vi "FRIC_navX_Internal_Serial_ProcessingLoop.vi"(9 "Stream Type":T1, 10 "Serial Port":T2, 11 "Update Rate (4Hz-100Hz)":u8=50 min=4 max=100) -> (0 "error out":errorcluster)   [LabVIEW 2015]
doc: "This navX VI handles the reading/writing for the navX. All of the good stuff is in here.\nTHIS VI SHOULD NOT BE CALLED BY THE USER!"
uses:
  navX Library v2/_TypeDefs/Z900_navX_DeviceTypeDef.ctl
  navX Library v2/_TypeDefs/Z900_navX_ProtocolTypeDef.ctl
  navX Library v2/_TypeDefs/Z900_navX_NotifyPacketTypeDef.ctl
  navX Library v2/_TypeDefs/Z900_navX_ActionTypeDef.ctl
  _NI WPI Serial USB/WPI_SerialPort_USB.ctl
  navX Library v2/_TypeDefs/Z900_navX_SerialStreamTypeDef.ctl
  TypeDefs/FRIC_navX_ProcessingLoopStatesTypeDef_I2C.ctl
  TypeDefs/FRIC_navX_I2C Process Loop TypeDef.ctl
  <vilib>/Rock Robotics/SystemInterfaces/Typedef/FPGA_TypedefDigitalModule.ctl
  <vilib>/Rock Robotics/SystemInterfaces/i2clib/i2c_bus.ctl
  navX Library v2/_TypeDefs/Z900_navX_IntegrationControlRegisters.ctl
  <vilib>/Rock Robotics/WPI/SPI/WPI_SPIDevRef.ctl
  <vilib>/Rock Robotics/SystemInterfaces/spilib/spi_bus.ctl
  <vilib>/Rock Robotics/WPI/SerialPort/WPI_SerialPortRef.ctl
  navX Library v2/_TypeDefs/Flags/Z900_navX_Flags_CapabilityTypeDef.ctl
  navX Library v2/_TypeDefs/Z900_navX_DeviceRegisters.ctl
  navX Library v2/_TypeDefs/navX Open TypeDefs/Z900_navX_OpenTypeDef_Serial.ctl
  navX Library v2/_Util/Encode Protocol/Z900_navX_Util_EncodeProtocol_SignedHundredths.vi
  navX Library v2/_Util/Encode Protocol/Z900_navX_Util_EncodeProtocol_UnsignedHundredths.vi
  navX Library v2/_Util/Encode Protocol/Z900_navX_Util_EncodeProtocol_UInt16.vi
  navX Library v2/Device/_Internal/SERIAL/Z900_navX_SERIAL_ValidatePacketChecksum.vi
  navX Library v2/Device/_Internal/SERIAL/Z900_navX_SERIAL_ValidatePacketTermination.vi
  navX Library v2/_Util/Encode Protocol/Z900_navX_Util_EncodeProtocol_Int16.vi
  navX Library v2/_Util/Z900_navX_Util_BigEndian_to_LittleEndian.vi
  <vilib>/Rock Robotics/SystemInterfaces/Utilities/FPGA_UtilitiesRead LocalTime.vi
  navX Library v2/navX Library v2.lvlib
  _NI WPI Serial USB/_NI WPI Serial USB.lvlib
panel:
  out "output cluster":T3={"Interface"={"Protocol"=enum."SERIAL", "Update Rate (4Hz-100Hz)"=4, "navX Open TypeDef"=variant}, "Notify Packet"=refnum, "Loop VI Refnum"=refnum, "Ready to Close Occurrence Refnum"=refnum, "Name"=""} {"Interface"."Update Rate (4Hz-100Hz)" min=4 max=60 step=1}
  out "Connected":bool
  in  "Halt":bool
  out "Registry":u8[](array[numeric])
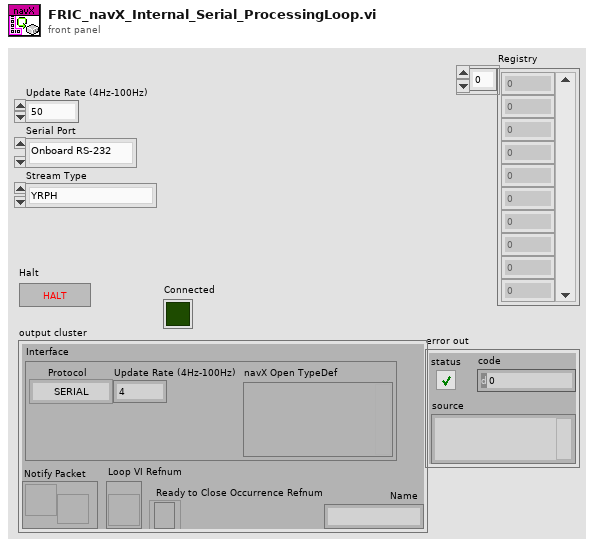
[diagram p1: front panel]
types:
  T1 = typedef "navX Library v2.lvlib/Z900_navX_SerialStreamTypeDef.ctl" = enum16{"YRPH", "Quaterinons", "Gyro/Raw", "AHRS", "AHRSAndPositioning"}
  T2 = typedef "_NI WPI Serial USB.lvlib/WPI_SerialPort_USB.ctl" = enum16{"Onboard RS-232", "MXP TTL", "USB"}
  T3 = typedef "navX Library v2.lvlib/Z900_navX_DeviceTypeDef.ctl" = cluster{"Interface":cluster{"Protocol":T4, "Update Rate (4Hz-100Hz)":u8, "navX Open TypeDef":variant}, "Notify Packet":refnum<notifier>, "Loop VI Refnum":refnum<vi>, "Ready to Close Occurrence Refnum":refnum<k4>, "Name":string}
  T4 = typedef "navX Library v2.lvlib/Z900_navX_ProtocolTypeDef.ctl" = enum16{"SERIAL", "I2C", "SPI"}
  T5 = typedef "FRIC_navX_ProcessingLoopStatesTypeDef_I2C.ctl" = enum16{"Process", "INI", "Check Packets Valid", "Close", "Decode Serial Packet", "Flush Serial", "Generate Command", "Last Packet Valid", "Open", "Read", "Reset Serial", "Set Termination Char", "Wait", "Write", "Exit"}
  T6 = typedef "FRIC_navX_I2C Process Loop TypeDef.ctl" = cluster{"State Array":T5[], "error":errorcluster, "FPGA Cluster":cluster{"Last Valid FPGA Time":dbl, "Error Count":i32, "Initialized":bool}, "Device Info":T3, "I2CDevRef":cluster{"DevStatus":errorcluster, "Controller":T7, "Device Address":u8, "Handle":i32, "I2C Bus":T8}, "Registry":u8[], "Command Array":T9[], "Connected?":bool, "navX Device Memory Size":i32, "notification":T10, "Memory Size Set":bool, "SPIDevRef":T12, "navX Serial Open":cluster{"Serial Port":T2, "Stream Type":T1}, "SerialPortRef":T14, "Serial Read Buffer":string, "Serial Write Buffer":string[]}
  T7 = typedef "FPGA_TypedefDigitalModule.ctl" = enum16{"Controller 1"}
  T8 = typedef "i2c_bus.ctl" = enum16{"I2C On-Board", "I2C MXP", "Invalid"}
  T9 = typedef "navX Library v2.lvlib/Z900_navX_IntegrationControlRegisters.ctl" = u8
  T10 = typedef "navX Library v2.lvlib/Z900_navX_NotifyPacketTypeDef.ctl" = cluster{"navX Action":T11, "Data":variant}
  T11 = typedef "navX Library v2.lvlib/Z900_navX_ActionTypeDef.ctl" = enum16{"None", "Halt", "Normal Read", "Update Serial Protocol", "Update Rate Htz", "Zero-Yaw", "Zero-Displacement", "Zero-Velocity"}
  T12 = typedef "WPI_SPIDevRef.ctl" = cluster{"DevStatus":errorcluster, "Handle":i32, "Controller":T7, "SPI Bus":T13}
  T13 = typedef "spi_bus.ctl" = enum16{"SPI On-Board, CS0", "SPI On-Board, CS1", "SPI On-Board, CS2", "SPI On-Board, CS3", "SPI MXP", "Invalid"}
  T14 = typedef "WPI_SerialPortRef.ctl" = cluster{"DevStatus":errorcluster, "Serial Port Name":refnum<visa-resource-name>}
  T15 = typedef "navX Library v2.lvlib/Z900_navX_OpenTypeDef_Serial.ctl" = cluster{"Serial Port":T2, "Stream Type":T1}
  T16 = typedef "navX Library v2.lvlib/Z900_navX_DeviceRegisters.ctl" = u8
  T17 = typedef "navX Library v2.lvlib/Z900_navX_Flags_CapabilityTypeDef.ctl" = u16
  T18 = cluster{"Last Valid FPGA Time":dbl, "Error Count":i32, "Initialized":bool}
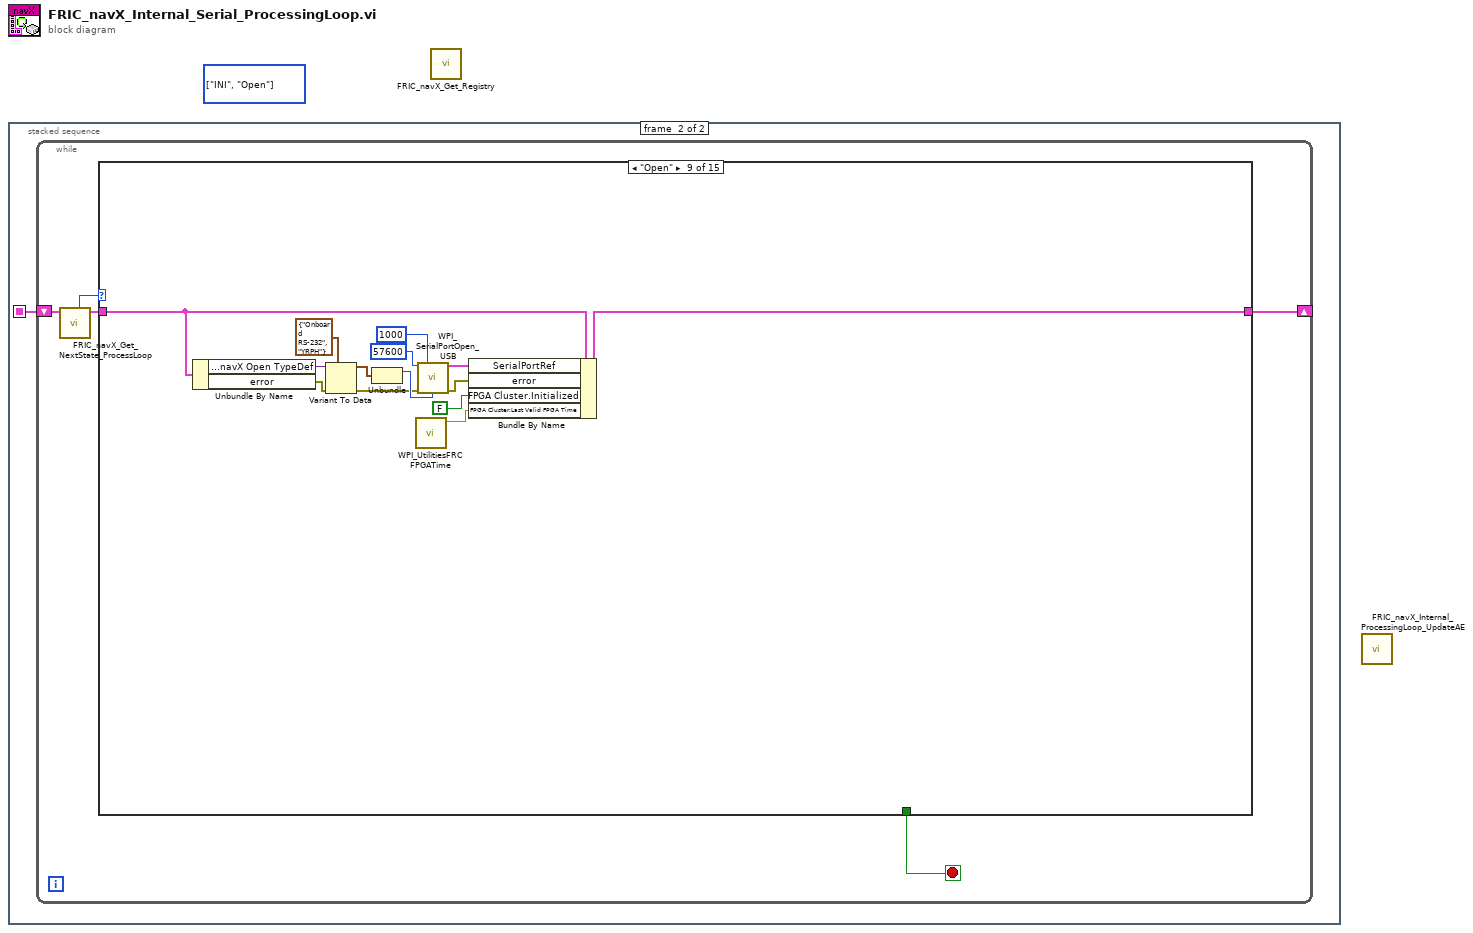
[diagram p0: block diagram]
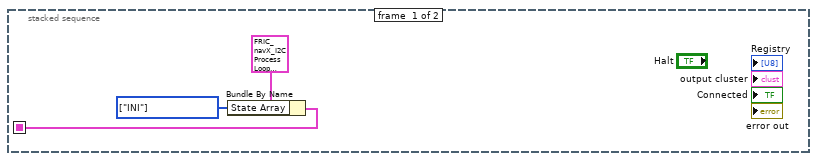
[diagram p2: hidden frame]
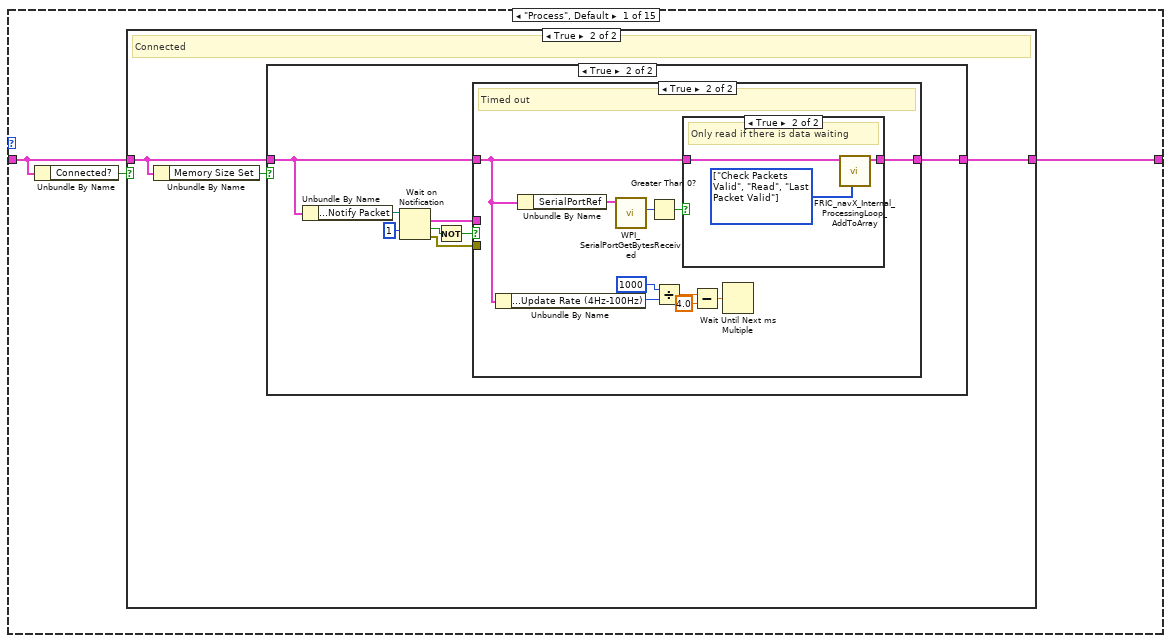
[diagram p3: hidden frame]
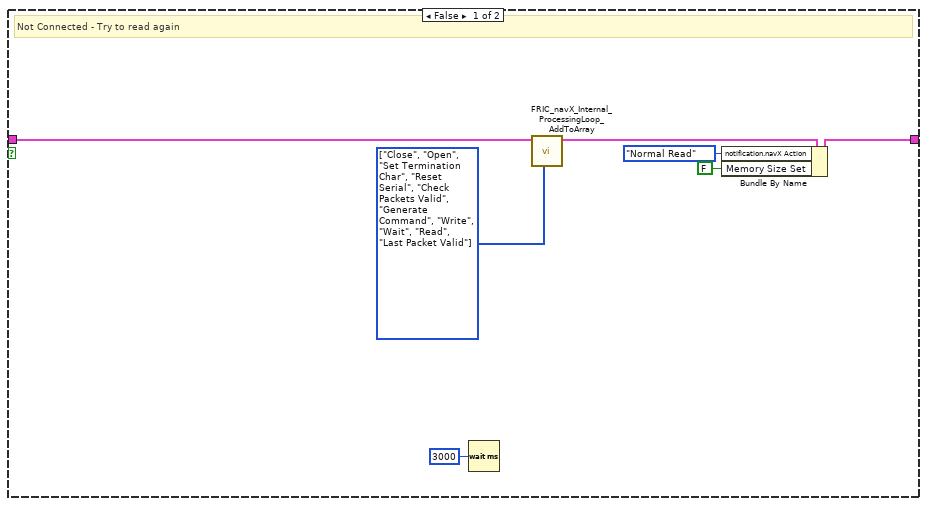
[diagram p4: hidden frame]
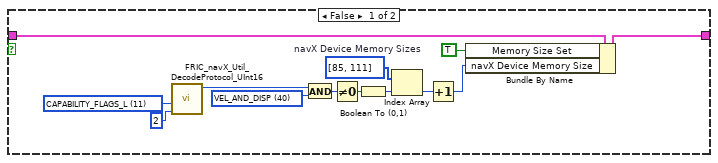
[diagram p5: hidden frame]
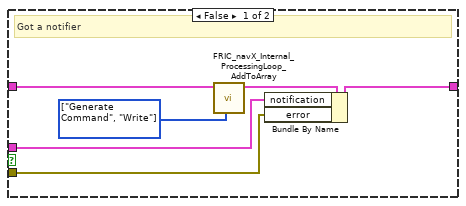
[diagram p6: hidden frame]
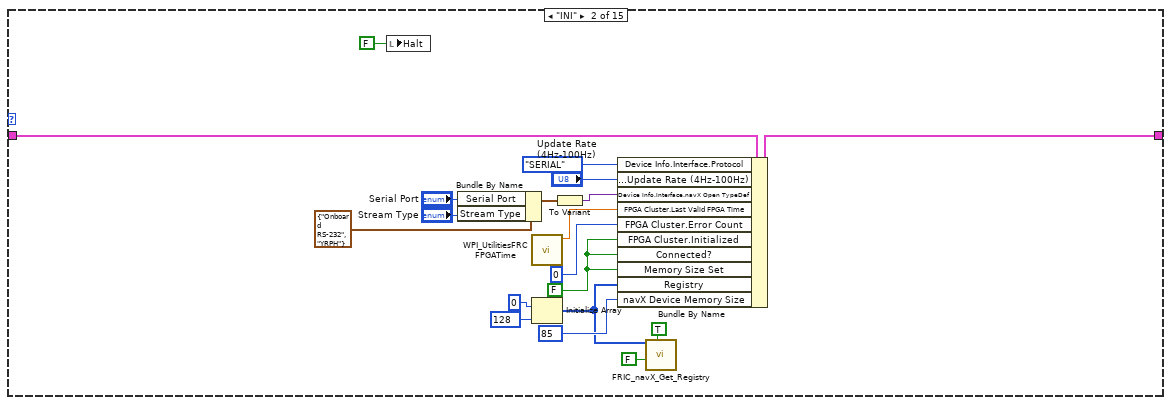
[diagram p8: hidden frame]
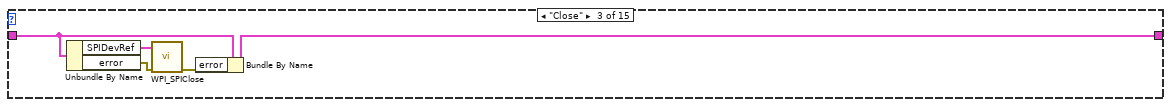
[diagram p9: hidden frame]
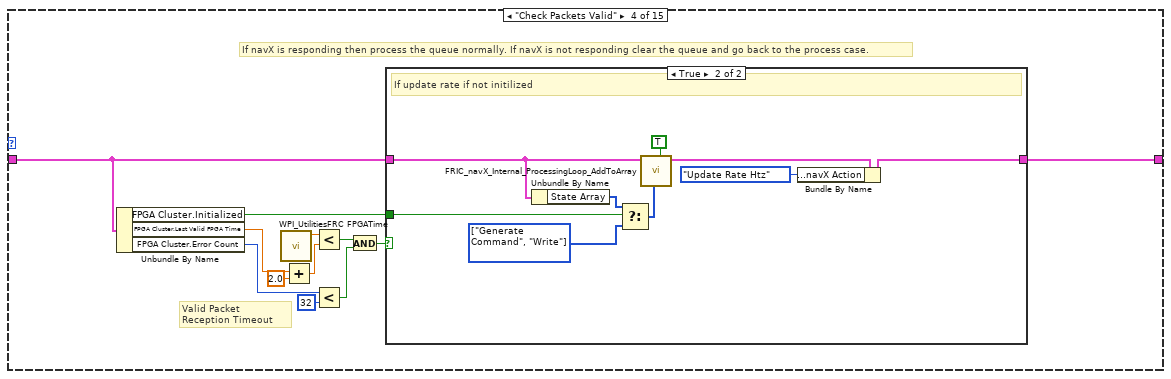
[diagram p10: hidden frame]
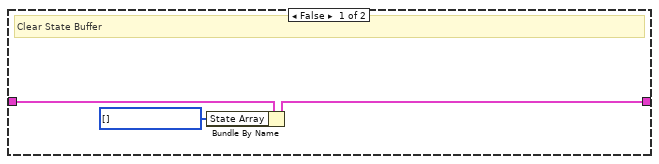
[diagram p11: hidden frame]
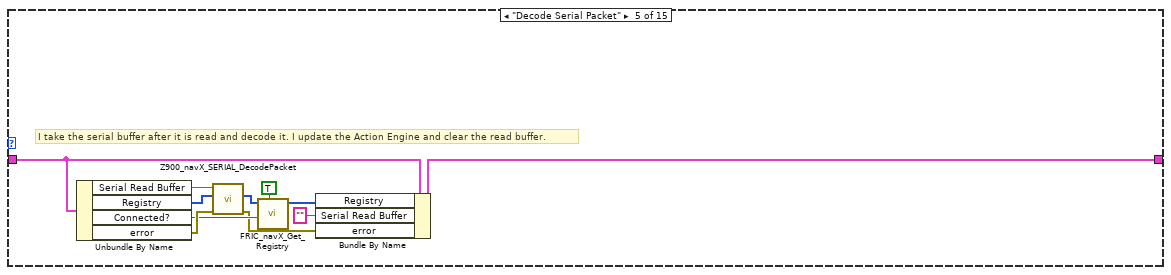
[diagram p12: hidden frame]
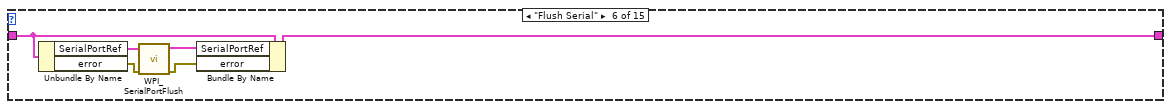
[diagram p13: hidden frame]
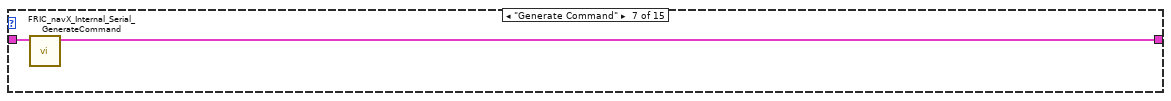
[diagram p14: hidden frame]
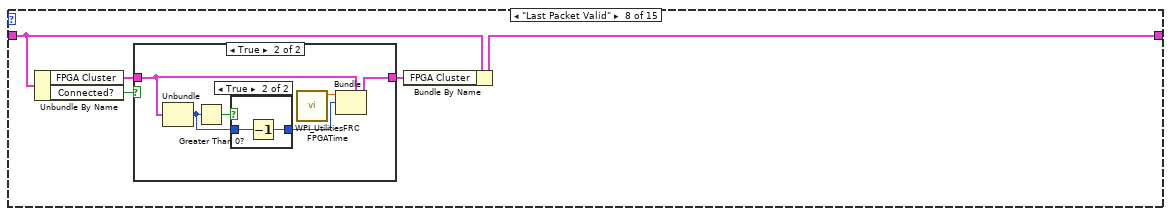
[diagram p15: hidden frame]
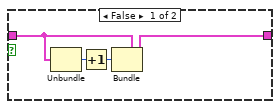
[diagram p16: hidden frame]
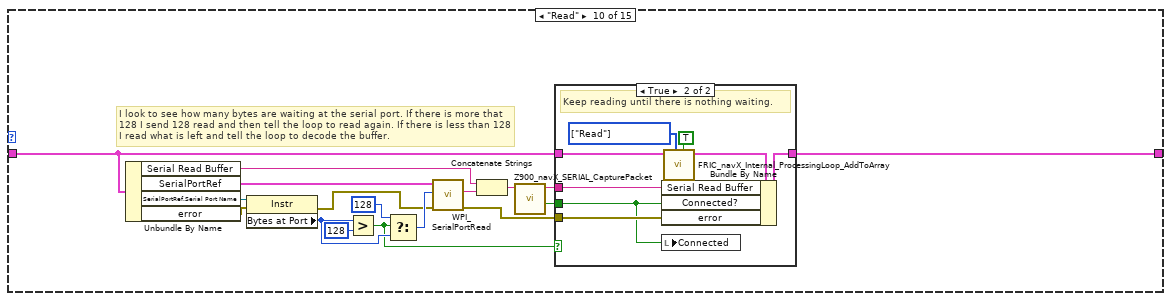
[diagram p18: hidden frame]
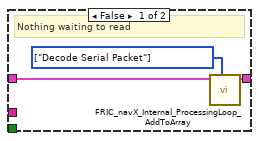
[diagram p19: hidden frame]
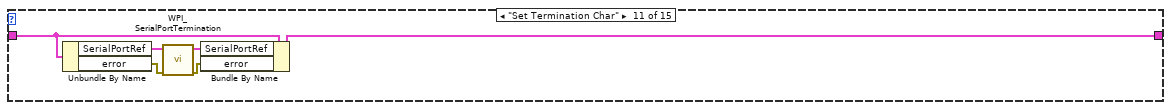
[diagram p20: hidden frame]
diagram:
  (unwired) T5[] [enum."INI", enum."Open"] items=["Process", "INI", "Check Packets Valid", "Close", "Decode Serial Packet", "Flush Serial", "Generate Command", "Last Packet Valid", "Open", "Read", "Reset Serial", "Set Termination Char", "Wait", "Write", "Exit"]
  n1 = stacked-sequence {
    seq-local: [w3 _] -> [_ w4]
    frame #0 {
      w1 = T5[] [enum."INI"] items=["Process", "INI", "Check Packets Valid", "Close", "Decode Serial Packet", "Flush Serial", "Generate Command", "Last Packet Valid", "Open", "Read", "Reset Serial", "Set Termination Char", "Wait", "Write", "Exit"] ("State Array")
      n2 = Bundle By Name(cluster=T6 {"State Array"=[enum."INI", enum."Open"], "error"={"status"=FALSE, "code"=0, "source"=""}, "FPGA Cluster"={"Last Valid FPGA Time"=0.0, "Error Count"=0, "Initialized"=FALSE}, "Device Info"={"Interface"={"Protocol"=enum."SERIAL", "Update Rate (4Hz-100Hz)"=4, "navX Open TypeDef"=variant}, "Notify Packet"=refnum, "Loop VI Refnum"=refnum, "Ready to Close Occurrence Refnum"=refnum, "Name"=""}, "I2CDevRef"={"DevStatus"={"status"=FALSE, "code"=0, "source"=""}, "Controller"=enum."Controller 1", "Device Address"=0, "Handle"=0, "I2C Bus"=enum."Invalid"}, "Registry"=[], "Command Array"=[214, 32], "Connected?"=FALSE, "navX Device Memory Size"=85, "notification"={"navX Action"=enum."None", "Data"=variant}, "Memory Size Set"=FALSE, "SPIDevRef"={"DevStatus"={"status"=FALSE, "code"=0, "source"=""}, "Handle"=0, "Controller"=enum."Controller 1", "SPI Bus"=enum."SPI On-Board, CS0"}, "navX Serial Open"={"Serial Port"=enum."Onboard RS-232", "Stream Type"=enum."YRPH"}, "SerialPortRef"={"DevStatus"={"status"=FALSE, "code"=0, "source"=""}, "Serial Port Name"=""}, "Serial Read Buffer"="", "Serial Write Buffer"=[]} ("I2C Process Loop TypeDef"), "State Array"=w1) -> (w3:T6)
    }
    frame #1 {
      n3 = while {
        shift-right: [w5] -> _
        shift-left: w4 -> [w8]
        stop <- w9 stop-if-true
        n4 = call "FRIC_navX_Get_NextState_ProcessLoop.vi"("I2C Process Loop TypeDef (in)"=w8) -> ("I2C Process Loop TypeDef (out)"=w7:T6, "Current State"=w6:T5)  [unwired: 9 in]
        n5 = case shown="\"Open\"" w6 {
          tunnel: [_ _ _ _ _ _ _ _ _ _ _ _ _ _ TRUE] -> w9
          tunnel: w7 -> [w10 w78 w87 w91 w117 w124 w130 w134 w160 w167 w191 w201 w204 w219 w226]
          tunnel: [w12 w72 w86 w92 w116 w123 w129 w133 w159 w166 w192 w202 w204 w207 w226] -> w5
          frame "Process", Default {
            n6 = Unbundle By Name(w10) -> ("Connected?"=w11:bool)
            n7 = case shown="True" w11 {
              tunnel: w10 -> [w18 w21]
              tunnel: [w15 w22] -> w12
              frame False {
                w17 = T5[] [enum."Close", enum."Open", enum."Set Termination Char", enum."Reset Serial", enum."Check Packets Valid", enum."Generate Command", enum."Write", enum."Wait", enum."Read", enum."Last Packet Valid"] items=["Process", "INI", "Check Packets Valid", "Close", "Decode Serial Packet", "Flush Serial", "Generate Command", "Last Packet Valid", "Open", "Read", "Reset Serial", "Set Termination Char", "Wait", "Write", "Exit"]
                # "Not Connected - Try to read again"
                n8 = Wait (ms)(milliseconds to wait=u32 3000) -> ()  [unwired: 1 out]
                n9 = call "FRIC_navX_Internal_ProcessingLoop_AddToArray.vi"("States Array"=w17, "I2C Process Loop TypeDef (in)"=w18) -> ("I2C Process Loop TypeDef (out)"=w16:T6)  [unwired: 9 in]
                n10 = Bundle By Name(cluster=w16, "notification.navX Action"=Z900_navX_ActionTypeDef."Normal Read", "Memory Size Set"=FALSE) -> (w15:T6)
              }
              frame True {
                # "Connected"
                n11 = Unbundle By Name(w21) -> ("Memory Size Set"=w20:bool)
                n12 = case shown="True" w20 {
                  tunnel: [w34 w40] -> w22
                  tunnel: w21 -> [w35 w36]
                  frame False {
                    w33 = T16 11 items=["WHOAMI"=0, "HW_REV"=1, "FW_VER_MAJOR"=2, "FW_VER_MINOR"=3, "UPDATE_RATE_HZ"=4, "ACCEL_FSR_G"=5, "GYRO_FSR_DPS"=6, "OP_STATUS"=8, "CAL_STATUS"=9, "SELFTEST_STATUS"=10, "CAPABILITY_FLAGS_L"=11, "CAPABILITY_FLAGS_H"=12, "SENSOR_STATUS"=16, "TIMESTAMP"=18, "YAW"=22, "ROLL"=24, "PITCH"=26, "HEADING"=28, "FUSED_HEADING"=30, "ALTITUDE_I"=32, "ALTITUDE_D"=34, "LINERA_ACC_X"=36, "LINERA_ACC_Y"=38, "LINERA_ACC_Z"=40, "QUAT_W"=42, "QUAT_X"=44, "QUAT_Y"=46, "QUAT_Z"=48, "MPU_TEMP_C"=50, "GYRO_X"=52, "GYRO_Y"=54, "GYRO_Z"=56, "ACC_X"=58, "ACC_Y"=60, "ACC_Z"=62, "MAG_X"=64, "MAG_Y"=66, "MAG_Z"=68, "PRESSURE_I"=70, "PRESSURE_D"=72, "PRESSURE_TEMP"=74, "YAW_OFFSET"=76, "QUAT_OFFSET_W"=78, "QUAT_OFFSET_X"=80, "QUAT_OFFSET_Y"=82, "QUAT_OFFSET_Z"=84, "INTEGRATION_CONTROL"=86, "VELOCITY_X"=88, "VELOCITY_Y"=92, "VELOCITY_Z"=96, "DISPLACMENT_X"=100, "DISPLACMENT_Y"=104, "DISPLACEMENT_Z"=108] ("Device Register")
                    w28 = T17 40 items=["OMNIMOUNT"=4, "OMNIMOUNT_CONFIG_MASK"=38, "VEL_AND_DISP"=40, "YAW_RESET"=80] ("Capability Flag")
                    w29 = i32[] [85, 111]  # navX Device Memory Sizes
                    n13 = call "FRIC_navX_Util_DecodeProtocol_UInt16.vi"("length"=2, "Device Register"=w33) -> ("Value"=w26:u16)  [unwired: 9 in]
                    n14 = And(x=w26, y=w28) -> (x .and. y?=w27:T17)
                    n15 = Not Equal To 0?(x=w27) -> (x != 0?=w30:bool)
                    n16 = Boolean To (0,1)(Boolean=w30) -> (0, 1=w31:i16)
                    n17 = Index Array(array=w29, index=w31) -> (element=w24:i32)
                    n18 = Increment(x=w24) -> (x+1=w23:i32)
                    n19 = Bundle By Name(cluster=w35, "Memory Size Set"=TRUE, "navX Device Memory Size"=w23) -> (w34:T6)
                  }
                  frame True {
                    n20 = Unbundle By Name(w36) -> ("Device Info.Notify Packet"=w43:refnum<notifier>)
                    n21 = Wait on Notification(notifier=w43, timeout in ms (-1)=1) -> (notification=w38:T10, timed out?=w41:bool, error out=w37:errorcluster)  [unwired: 2 in, 1 out]
                    n22 = Not(x=w41) -> (.not. x?=w39:bool)
                    n23 = case shown="True" w39 {
                      tunnel: w36 -> [w49 w53]
                      tunnel: [w48 w54] -> w40
                      tunnel: w38 -> [w47 _]
                      tunnel: w37 -> [w44 _]
                      frame False {
                        w45 = T5[] [enum."Generate Command", enum."Write"] items=["Process", "INI", "Check Packets Valid", "Close", "Decode Serial Packet", "Flush Serial", "Generate Command", "Last Packet Valid", "Open", "Read", "Reset Serial", "Set Termination Char", "Wait", "Write", "Exit"] ("States Array")
                        # "Got a notifier"
                        n24 = call "FRIC_navX_Internal_ProcessingLoop_AddToArray.vi"("States Array"=w45, "I2C Process Loop TypeDef (in)"=w49) -> ("I2C Process Loop TypeDef (out)"=w46:T6)  [unwired: 9 in]
                        n25 = Bundle By Name(cluster=w46, "notification"=w47, "error"=w44) -> (w48:T6)
                      }
                      frame True {
                        # "Timed out"
                        n26 = Unbundle By Name(w53) -> ("Device Info.Interface.Update Rate (4Hz-100Hz)"=w59:u8)
                        n27 = Unbundle By Name(w53) -> ("SerialPortRef"=w52:T14)
                        n28 = call <vilib>:"WPI_SerialPortGetBytesReceived.vi"("SerialPortRef"=w52) -> ("Bytes at Port"=w51:u32)  [unwired: 8 in, 2 out]
                        n29 = Greater Than 0?(x=w51) -> (x > 0?=w50:bool)
                        n30 = Divide(x=i16 1000, y=w59) -> (x/y=w57:dbl)
                        n31 = case shown="True" w50 {
                          tunnel: [w60 w62] -> w54
                          tunnel: w53 -> [w60 w61]
                          frame False {
                          }
                          frame True {
                            w63 = T5[] [enum."Check Packets Valid", enum."Read", enum."Last Packet Valid"] items=["Process", "INI", "Check Packets Valid", "Close", "Decode Serial Packet", "Flush Serial", "Generate Command", "Last Packet Valid", "Open", "Read", "Reset Serial", "Set Termination Char", "Wait", "Write", "Exit"]
                            # "Only read if there is data waiting"
                            n32 = call "FRIC_navX_Internal_ProcessingLoop_AddToArray.vi"("States Array"=w63, "I2C Process Loop TypeDef (in)"=w61) -> ("I2C Process Loop TypeDef (out)"=w62:T6)  [unwired: 9 in]
                          }
                        }
                        n33 = Subtract(x=w57, y=4.0) -> (x-y=w55:dbl)
                        n34 = Wait Until Next ms Multiple(millisecond multiple=w55) -> ()  [unwired: 1 out]
                      }
                    }
                  }
                }
              }
            }
          }
          frame "INI" {
            w70 = FALSE ("Initialized")
            n35 = local write "Halt"(FALSE ("Halt")) -> ()
            n36 = Bundle By Name(cluster=T15 {"Serial Port"=enum."Onboard RS-232", "Stream Type"=enum."YRPH"} ("navX Serial Open"), "Serial Port"="Serial Port", "Stream Type"="Stream Type") -> (w79:T15)
            n37 = call <vilib>:"WPI_UtilitiesFRC FPGATime.vi"() -> ("FPGA Time"=w74:dbl)  [unwired: 10 in, 1 out]
            n38 = Initialize Array(u8 0 ("Received Data"), 128 ("hex")) -> (w68:u8[])
            n39 = To Variant(anything=w79) -> (Variant=w75:variant)
            n40 = Bundle By Name(cluster=w78, "Device Info.Interface.Protocol"=Z900_navX_ProtocolTypeDef."SERIAL" ("Protocol"), "Device Info.Interface.Update Rate (4Hz-100Hz)"="Update Rate (4Hz-100Hz)", "Device Info.Interface.navX Open TypeDef"=w75, "FPGA Cluster.Last Valid FPGA Time"=w74, "FPGA Cluster.Error Count"=0 ("Error Count"), "FPGA Cluster.Initialized"=w70, "Connected?"=w70, "Memory Size Set"=w70, "Registry"=w68, "navX Device Memory Size"=85 ("hex")) -> (w72:T6)
            n41 = call "FRIC_navX_Get_Registry.vi"("Update"=TRUE, "Connected?"=FALSE, "Registry (in)"=w68) -> ()  [unwired: 7 in, 2 out]
          }
          frame "Close" {
            n42 = Unbundle By Name(w87) -> ("SPIDevRef"=w85:T12, "error"=w84:errorcluster)
            n43 = call <vilib>:"WPI_SPIClose.vi"("error in (no error)"=w84, "SPIDevRef"=w85) -> ("error out"=w83:errorcluster)  [unwired: 9 in]
            n44 = Bundle By Name(cluster=w87, "error"=w83) -> (w86:T6)
          }
          frame "Check Packets Valid" {
            # "If navX is responding then process the queue normally. If navX is not responding clear the queue and go back to the process case."
            # "Valid Packet Reception Timeout"
            n45 = Unbundle By Name(w91) -> ("FPGA Cluster.Initialized"=w89:bool, "FPGA Cluster.Last Valid FPGA Time"=w90:dbl, "FPGA Cluster.Error Count"=w88:i32)
            n46 = call <vilib>:"WPI_UtilitiesFRC FPGATime.vi"() -> ("FPGA Time"=w97:dbl)  [unwired: 10 in, 1 out]
            n47 = Add(x=w90, y=2.0) -> (x+y=w98:dbl)
            n48 = Less?(x=w97, y=w98) -> (x < y?=w95:bool)
            n49 = Less?(x=w88, y=32) -> (x < y?=w94:bool)
            n50 = And(x=w95, y=w94) -> (x .and. y?=w93:bool)
            n51 = case shown="True" w93 {
              tunnel: w91 -> [w102 w109]
              tunnel: [w101 w104] -> w92
              tunnel: w89 -> [_ w110]
              frame False {
                w100 = T5[] [] items=["Process", "INI", "Check Packets Valid", "Close", "Decode Serial Packet", "Flush Serial", "Generate Command", "Last Packet Valid", "Open", "Read", "Reset Serial", "Set Termination Char", "Wait", "Write", "Exit"] ("f")
                # "Clear State Buffer"
                n52 = Bundle By Name(cluster=w102, "State Array"=w100) -> (w101:T6)
              }
              frame True {
                w106 = T5[] [enum."Generate Command", enum."Write"] items=["Process", "INI", "Check Packets Valid", "Close", "Decode Serial Packet", "Flush Serial", "Generate Command", "Last Packet Valid", "Open", "Read", "Reset Serial", "Set Termination Char", "Wait", "Write", "Exit"] ("f")
                # "If update rate if not initilized"
                n53 = Unbundle By Name(w109) -> ("State Array"=w108:T5[])
                n54 = Select(t=w108, s=w110, f=w106) -> (s? t:f=w107:T5[])
                n55 = call "FRIC_navX_Internal_ProcessingLoop_AddToArray.vi"("Add to beginning"=TRUE, "States Array"=w107, "I2C Process Loop TypeDef (in)"=w109) -> ("I2C Process Loop TypeDef (out)"=w105:T6)  [unwired: 8 in]
                n56 = Bundle By Name(cluster=w105, "notification.navX Action"=Z900_navX_ActionTypeDef."Update Rate Htz") -> (w104:T6)
              }
            }
          }
          frame "Decode Serial Packet" {
            # "I take the serial buffer after it is read and decode it. I update the Action Engine and clear the read buffer."
            n57 = Unbundle By Name(w117) -> ("Serial Read Buffer"=w120:string, "Registry"=w119:u8[], "Connected?"=w113:bool, "error"=w114:errorcluster)
            n58 = call "Z900_navX_SERIAL_DecodePacket.vi"("error in (no error)"=w114, "Data"=w119, "Packet"=w120) -> ("error out"=w112:errorcluster, "Data"=w118:u8[])  [unwired: 6 in, 1 out]
            n59 = call "FRIC_navX_Get_Registry.vi"("Update"=TRUE, "Connected?"=w113, "Registry (in)"=w118) -> ("Registry (out)"=w121:u8[])  [unwired: 7 in, 1 out]
            n60 = Bundle By Name(cluster=w117, "Registry"=w121, "Serial Read Buffer"="", "error"=w112) -> (w116:T6)
          }
          frame "Flush Serial" {
            n61 = Unbundle By Name(w124) -> ("SerialPortRef"=w128:T14, "error"=w127:errorcluster)
            n62 = call <vilib>:"WPI_SerialPortFlush.vi"("error in (no error)"=w127, "SerialPortRef"=w128) -> ("error out"=w125:errorcluster, "SerialPortRef"=w126:T14)  [unwired: 8 in]
            n63 = Bundle By Name(cluster=w124, "SerialPortRef"=w126, "error"=w125) -> (w123:T6)
          }
          frame "Generate Command" {
            n64 = call "FRIC_navX_Internal_Serial_GenerateCommand.vi"("I2C Process Loop TypeDef (in)"=w130) -> ("I2C Process Loop TypeDef (out)"=w129:T6)  [unwired: 10 in]
          }
          frame "Last Packet Valid" {
            n65 = Unbundle By Name(w134) -> ("FPGA Cluster"=w135:T18, "Connected?"=w131:bool)
            n66 = case shown="True" w131 {
              tunnel: [w138 w145] -> w132
              tunnel: w135 -> [w137 w141]
              frame False {
                n67 = Unbundle(w137) -> ("Error Count"=w136:i32)  [unwired: 2 out]
                n68 = Increment(x=w136) -> (x+1=w139:i32)
                n69 = Bundle(cluster=w137, "Error Count"=w139) -> (w138:T18)  [unwired: 2 in]
              }
              frame True {
                n70 = Unbundle(w141) -> ("Error Count"=w140:i32)  [unwired: 2 out]
                n71 = Greater Than 0?(x=w140) -> (x > 0?=w143:bool)
                n72 = case shown="True" w143 {
                  tunnel: [w146 w148] -> w142
                  tunnel: w140 -> [w146 w147]
                  frame False {
                  }
                  frame True {
                    n73 = Decrement(x=w147) -> (x-1=w148:i32)
                  }
                }
                n74 = call <vilib>:"WPI_UtilitiesFRC FPGATime.vi"() -> ("FPGA Time"=w144:dbl)  [unwired: 10 in, 1 out]
                n75 = Bundle(cluster=w141, "Last Valid FPGA Time"=w144, "Error Count"=w142) -> (w145:T18)  [unwired: 1 in]
              }
            }
            n76 = Bundle By Name(cluster=w134, "FPGA Cluster"=w132) -> (w133:T6)
          }
          frame "Open" {
            n77 = Unbundle By Name(w160) -> ("Device Info.Interface.navX Open TypeDef"=w162:variant, "error"=w158:errorcluster)
            n78 = Variant To Data(error in=w158, type=T15 {"Serial Port"=enum."Onboard RS-232", "Stream Type"=enum."YRPH"} ("navX Serial Open"), Variant=w162) -> (data=w161:T15, error out=w152:errorcluster)
            n79 = Unbundle(w161) -> ("Serial Port"=w153:T2)  [unwired: 1 out]
            n80 = call <vilib>:"WPI_UtilitiesFRC FPGATime.vi"() -> ("FPGA Time"=w149:dbl)  [unwired: 10 in, 1 out]
            n81 = call "WPI_SerialPortOpen_USB.vi"("Baud Rate"=u32 57600, "Timeout Value (ms)"=u32 1000, "error in (no error)"=w152, "Serial Port"=w153) -> ("SerialPortRef"=w150:T14, "error out"=w151:errorcluster)  [unwired: 10 in]
            n82 = Bundle By Name(cluster=w160, "SerialPortRef"=w150, "error"=w151, "FPGA Cluster.Initialized"=FALSE ("Initialized"), "FPGA Cluster.Last Valid FPGA Time"=w149) -> (w159:T6)
          }
          frame "Read" {
            # "I look to see how many bytes are waiting at the serial port. If there is more that 128 I send 128 read and then tell the loop to read again. If there is less than 128 I read what is left and tell the loop to decode the buffer."
            n83 = Unbundle By Name(w167) -> ("Serial Read Buffer"=w175:string, "SerialPortRef"=w176:T14, "SerialPortRef.Serial Port Name"=w179:refnum<visa-resource-name>, "error"=w178:errorcluster)
            n84 = property class="Instr"(reference=w179, error in=w178) -> (error out=w169:errorcluster, "Bytes at Port"=w172:u32)  [unwired: 1 in]
            n85 = Greater?(x=w172, y=u32 128) -> (0:w168:bool)
            n86 = Select(t=u32 128 ("y"), s=w168, f=w172) -> (s? t:f=w170:u32)
            n87 = call <vilib>:"WPI_SerialPortRead.vi"("error in (no error)"=w169, "Num Bytes to Read"=w170, "SerialPortRef"=w176) -> ("error out"=w163:errorcluster, "Buffer"=w177:string)  [unwired: 6 in, 1 out]
            n88 = Concatenate Strings(w175, w177) -> (w174:string)
            n89 = call "Z900_navX_SERIAL_CapturePacket.vi"("Buffer"=w174) -> ("Packet Located"=w164:bool, "Buffer"=w165:string)  [unwired: 7 in, 2 out]
            n90 = case shown="True" w168 {
              tunnel: w167 -> [w182 w190]
              tunnel: [w181 w186] -> w166
              tunnel: w165 -> [_ w185]
              tunnel: w164 -> [_ w183]
              tunnel: w163 -> [_ w184]
              frame False {
                w180 = T5[] [enum."Decode Serial Packet"] items=["Process", "INI", "Check Packets Valid", "Close", "Decode Serial Packet", "Flush Serial", "Generate Command", "Last Packet Valid", "Open", "Read", "Reset Serial", "Set Termination Char", "Wait", "Write", "Exit"] ("States Array")
                # "Nothing waiting to read"
                n91 = call "FRIC_navX_Internal_ProcessingLoop_AddToArray.vi"("States Array"=w180, "I2C Process Loop TypeDef (in)"=w182) -> ("I2C Process Loop TypeDef (out)"=w181:T6)  [unwired: 9 in]
              }
              frame True {
                w189 = T5[] [enum."Read"] items=["Process", "INI", "Check Packets Valid", "Close", "Decode Serial Packet", "Flush Serial", "Generate Command", "Last Packet Valid", "Open", "Read", "Reset Serial", "Set Termination Char", "Wait", "Write", "Exit"] ("States Array")
                # "Keep reading until there is nothing waiting."
                n92 = local write "Connected"(w183) -> ()
                n93 = call "FRIC_navX_Internal_ProcessingLoop_AddToArray.vi"("Add to beginning"=TRUE, "States Array"=w189, "I2C Process Loop TypeDef (in)"=w190) -> ("I2C Process Loop TypeDef (out)"=w187:T6)  [unwired: 8 in]
                n94 = Bundle By Name(cluster=w187, "Serial Read Buffer"=w185, "Connected?"=w183, "error"=w184) -> (w186:T6)
              }
            }
          }
          frame "Set Termination Char" {
            n95 = Unbundle By Name(w191) -> ("SerialPortRef"=w196:T14, "error"=w195:errorcluster)
            n96 = call <vilib>:"WPI_SerialPortTermination.vi"("error in (no error)"=w195, "SerialPortRef"=w196) -> ("error out"=w193:errorcluster, "SerialPortRef"=w194:T14)  [unwired: 8 in]
            n97 = Bundle By Name(cluster=w191, "SerialPortRef"=w194, "error"=w193) -> (w192:T6)
          }
          frame "Reset Serial" {
            n98 = Unbundle By Name(w201) -> ("SerialPortRef"=w200:T14, "error"=w198:errorcluster)
            n99 = call <vilib>:"WPI_SerialPortReset.vi"("error in (no error)"=w198, "SerialPortRef"=w200) -> ("error out"=w197:errorcluster, "SerialPortRef"=w199:T14)  [unwired: 8 in]
            n100 = Bundle By Name(cluster=w201, "SerialPortRef"=w199, "error"=w197) -> (w202:T6)
          }
          frame "Wait" {
            n101 = Wait (ms)(milliseconds to wait=u32 1) -> ()  [unwired: 1 out]
          }
          frame "Write" {
            w206 = T5[] [enum."Flush Serial"] items=["Process", "INI", "Check Packets Valid", "Close", "Decode Serial Packet", "Flush Serial", "Generate Command", "Last Packet Valid", "Open", "Read", "Reset Serial", "Set Termination Char", "Wait", "Write", "Exit"] ("States Array")
            # "This adds a flush after any write so we don't always have to tell the array to flush."
            n102 = Unbundle By Name(w219) -> ("SerialPortRef"=w217:T14, "Serial Write Buffer"=w214:string[], "SerialPortRef.DevStatus"=w218:errorcluster)
            n103 = Delete From Array(array=w214, index=0) -> (deleted portion=w213:string, array with subset deleted=w210:string[])  [unwired: 1 in]
            n104 = call <vilib>:"WPI_SerialPortWrite.vi"("error in (no error)"=w218, "Buffer"=w213, "SerialPortRef"=w217) -> ("error out"=w216:errorcluster, "SerialPortRef"=w215:T14)  [unwired: 6 in, 1 out]
            n105 = Empty Array?(array=w210) -> (empty?=w209:bool)
            n106 = Bundle By Name(cluster=w219, "SerialPortRef"=w215, "error"=w216, "Serial Write Buffer"=w210) -> (w211:T6)
            n107 = case shown="False" w209 {
              tunnel: [w223 w224] -> w208
              tunnel: w211 -> [w222 w224]
              frame False {
                w221 = T5[] [enum."Write"] items=["Process", "INI", "Check Packets Valid", "Close", "Decode Serial Packet", "Flush Serial", "Generate Command", "Last Packet Valid", "Open", "Read", "Reset Serial", "Set Termination Char", "Wait", "Write", "Exit"] ("States Array")
                # "Write again because buffer is not empty."
                n108 = call "FRIC_navX_Internal_ProcessingLoop_AddToArray.vi"("Add to beginning"=TRUE, "States Array"=w221, "I2C Process Loop TypeDef (in)"=w222) -> ("I2C Process Loop TypeDef (out)"=w223:T6)  [unwired: 8 in]
              }
              frame True {
                # "Process the rest of the state array"
              }
            }
            n109 = call "FRIC_navX_Internal_ProcessingLoop_AddToArray.vi"("Add to beginning"=TRUE, "States Array"=w206, "I2C Process Loop TypeDef (in)"=w208) -> ("I2C Process Loop TypeDef (out)"=w207:T6)  [unwired: 8 in]
          }
          frame "Exit" {
            n110 = Unbundle By Name(w226) -> ("Device Info"=w225:T3)
            n111 = in-place {
              in-place-border: [TRUE] -> w228
              in-place-border: w225 -> [w229]
              # "Set Occurence of Close"
              n112 = Unbundle By Name(w229) -> ("Ready to Close Occurrence Refnum"=w231:refnum<k4>)
              n113 = local write "Halt"(FALSE ("Halt")) -> ()
              n114 = Set Occurrence(w231) -> ()
            }
            n115 = Stop(stop? (T)=w228) -> ()
          }
        }
      }
    }
  }
  n116 = call "FRIC_navX_Get_Registry.vi"() -> ()  [unwired: 10 in, 2 out]
  n117 = call "FRIC_navX_Internal_ProcessingLoop_UpdateAE.vi"() -> ()  [unwired: 6 in, 10 out]
